vi "SW_Calc_speed_2.vi"(3 "Speed smoothing type":u16(ring)=3 items=["None", "Holoborodko 2/5", "Holoborodko 2/7", "Holoborodko 2/11", "Holoborodko 4/7"], 4 "X coord, mm":dbl, 5 "Y coord, mm":dbl, 6 "Time per frame, s":dbl) -> (2 "Mouse speed, mm/s":dbl)   [LabVIEW 2018]
doc: "This VI calculates speed using smoothing of the input noisy data according to Holoborodko' algorithm: http://www.holoborodko.com/pavel/numerical-methods/numerical-derivative/smooth-low-noise-differentiator"
panel:
  out "Mouse speed for saving, mm/s":string
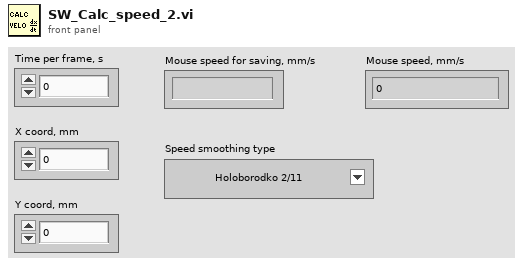
[diagram p1: front panel]
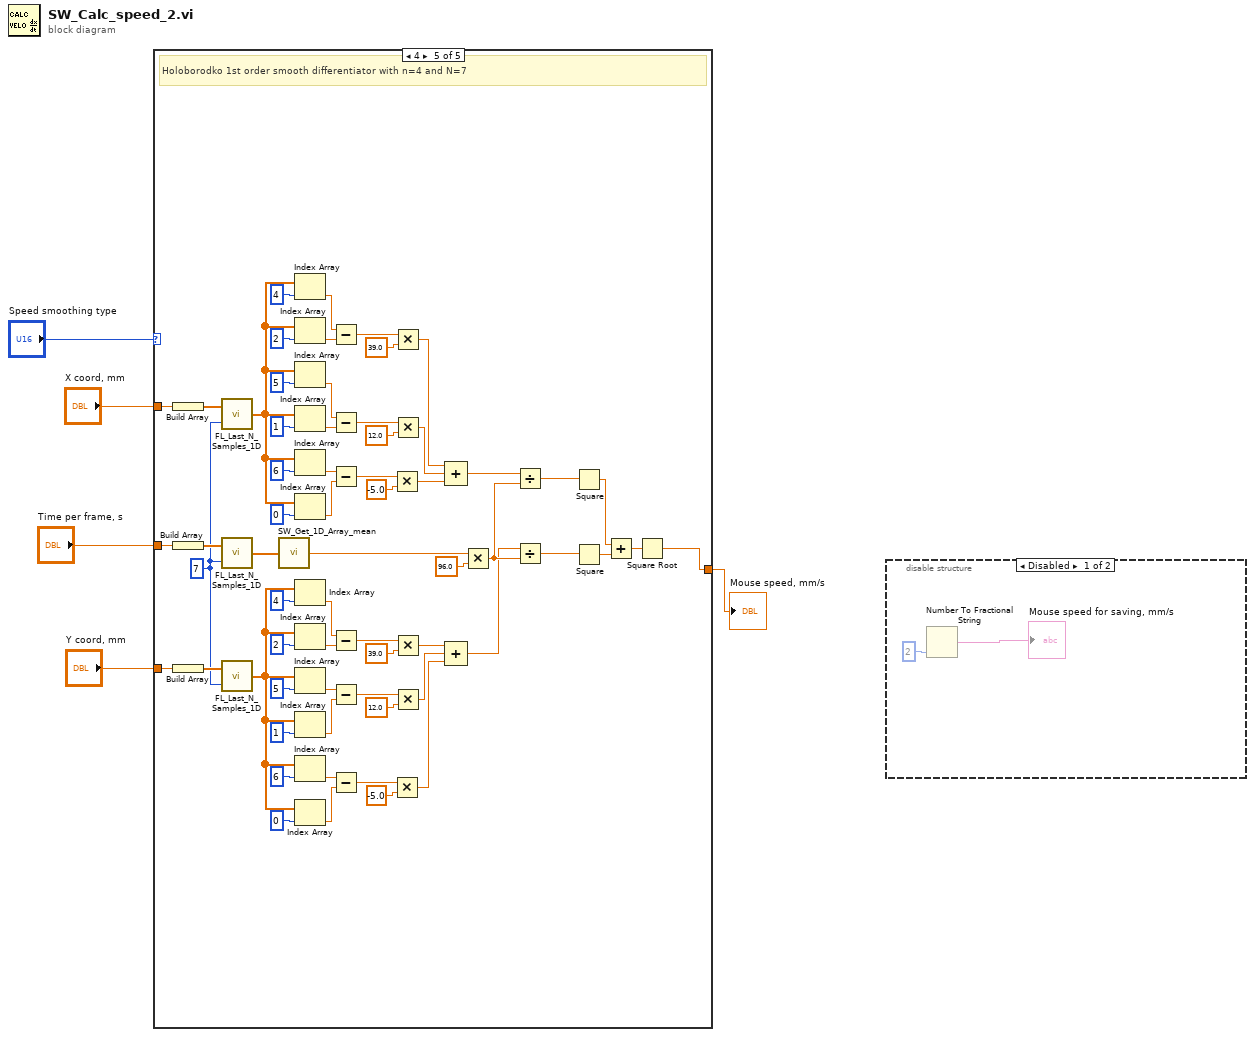
[diagram p0: block diagram]
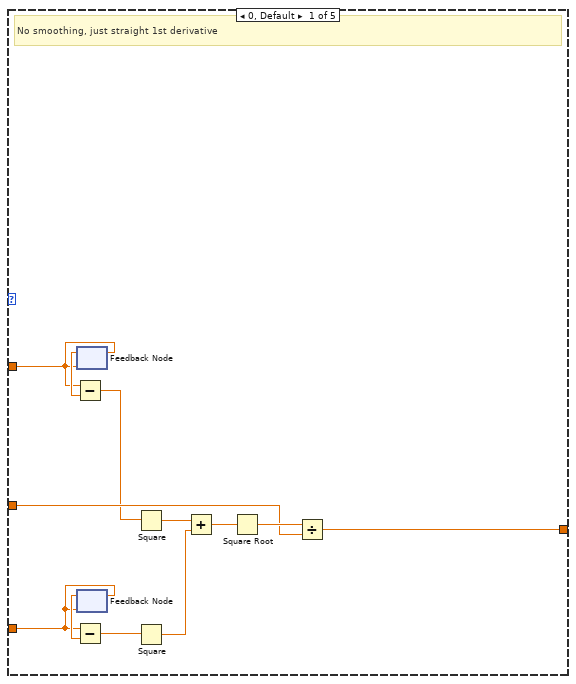
[diagram p3: hidden frame]
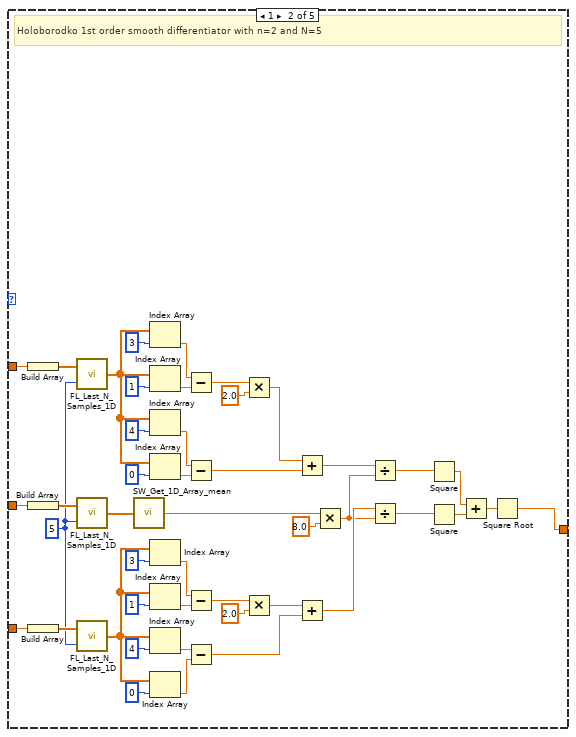
[diagram p4: hidden frame]
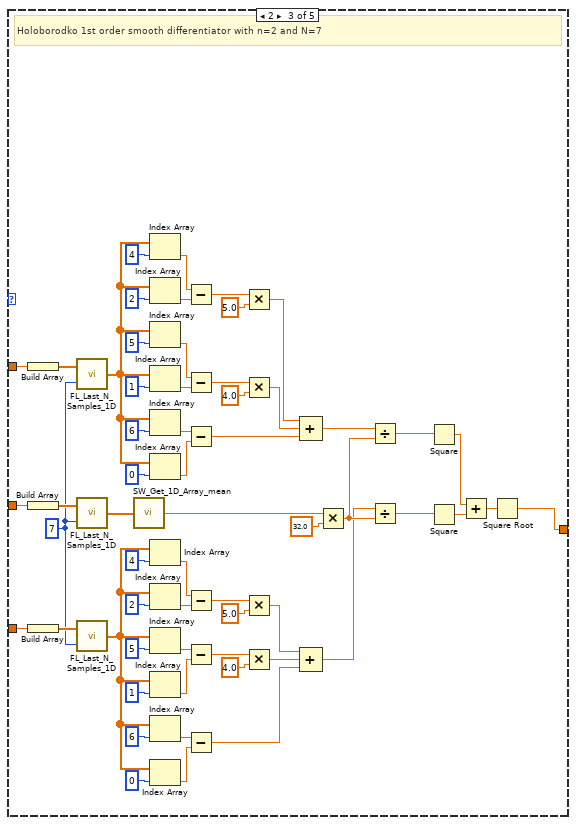
[diagram p5: hidden frame]
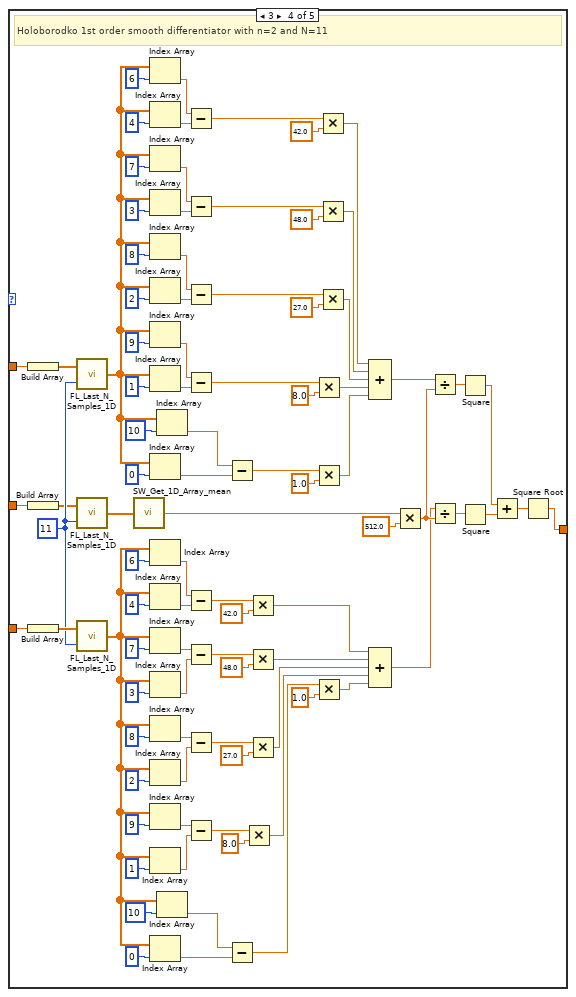
[diagram p6: hidden frame]
diagram:
  n1 = case shown="4" "Speed smoothing type" {
    tunnel: "Time per frame, s" -> [w13 w62 w121 w125 w275]
    tunnel: "Y coord, mm" -> [w7 w58 w117 w210 w271]
    tunnel: "X coord, mm" -> [w9 w57 w116 w209 w270]
    tunnel: [w12 w20 w99 w192 w253] -> w1
    frame 0, Default {
      # "No smoothing, just straight 1st derivative"
      n2 = feedback #1(w9) -> (w10:dbl)
      n3 = Subtract(x=w9, y=w10) -> (x-y=w8:dbl)
      n4 = feedback-in #1(w9) -> ()
      n5 = feedback #2(w7) -> (w11:dbl)
      n6 = Subtract(x=w7, y=w11) -> (x-y=w6:dbl)
      n7 = feedback-in #2(w7) -> ()
      n8 = Square(x=w8) -> (x^2=w16:dbl)
      n9 = Square(x=w6) -> (x^2=w17:dbl)
      n10 = Add(x=w16, y=w17) -> (x+y=w15:dbl)
      n11 = Square Root(x=w15) -> (sqrt(x)=w14:dbl)
      n12 = Divide(x=w14, y=w13) -> (x/y=w12:dbl)
    }
    frame 1 {
      w56 = u32 5 ("BufferLengthSamples")
      # "Holoborodko 1st order smooth differentiator with n=2 and N=5"
      n13 = Build Array(w57) -> (w60:dbl[])
      n14 = Build Array(w62) -> (w61:dbl[])
      n15 = Build Array(w58) -> (w59:dbl[])
      n16 = call "FL_Last_N_Samples_1D.vi"("BufferLengthSamples"=w56, "Input Array"=w60) -> ("Output Array"=w47:dbl[])
      n17 = call "FL_Last_N_Samples_1D.vi"("BufferLengthSamples"=w56, "Input Array"=w61) -> ("Output Array"=w19:dbl[])
      n18 = call "FL_Last_N_Samples_1D.vi"("BufferLengthSamples"=w56, "Input Array"=w59) -> ("Output Array"=w27:dbl[])
      n19 = call "SW_Get_1D_Array_mean.vi"("1D array"=w19) -> ("Mean of 1D Array"=w18:dbl)
      n20 = Index Array(array=w47, index=3) -> (element=w53:dbl)
      n21 = Index Array(array=w47, index=1) -> (element=w52:dbl)
      n22 = Index Array(array=w47, index=4) -> (element=w46:dbl)
      n23 = Index Array(array=w47, index=0) -> (element=w45:dbl)
      n24 = Index Array(array=w27, index=3) -> (element=w30:dbl)
      n25 = Index Array(array=w27, index=1) -> (element=w31:dbl)
      n26 = Index Array(array=w27, index=4) -> (element=w36:dbl)
      n27 = Index Array(array=w27, index=0) -> (element=w37:dbl)
      n28 = Subtract(x=w53, y=w52) -> (x-y=w51:dbl)
      n29 = Subtract(x=w46, y=w45) -> (x-y=w43:dbl)
      n30 = Subtract(x=w30, y=w31) -> (x-y=w32:dbl)
      n31 = Subtract(x=w36, y=w37) -> (x-y=w39:dbl)
      n32 = Multiply(x=w51, y=2.0) -> (x*y=w44:dbl)
      n33 = Multiply(x=w32, y=2.0) -> (x*y=w38:dbl)
      n34 = Add(x=w44, y=w43) -> (x+y=w42:dbl)
      n35 = Add(x=w38, y=w39) -> (x+y=w40:dbl)
      n36 = Multiply(x=w18, y=8.0) -> (x*y=w26:dbl)
      n37 = Divide(x=w42, y=w26) -> (x/y=w23:dbl)
      n38 = Divide(x=w40, y=w26) -> (x/y=w21:dbl)
      n39 = Square(x=w23) -> (x^2=w22:dbl)
      n40 = Square(x=w21) -> (x^2=w24:dbl)
      n41 = Add(x=w22, y=w24) -> (x+y=w25:dbl)
      n42 = Square Root(x=w25) -> (sqrt(x)=w20:dbl)
    }
    frame 2 {
      w115 = u32 7 ("BufferLengthSamples")
      # "Holoborodko 1st order smooth differentiator with n=2 and N=7"
      n43 = Build Array(w116) -> (w119:dbl[])
      n44 = Build Array(w121) -> (w120:dbl[])
      n45 = Build Array(w117) -> (w118:dbl[])
      n46 = call "FL_Last_N_Samples_1D.vi"("BufferLengthSamples"=w115, "Input Array"=w119) -> ("Output Array"=w94:dbl[])
      n47 = call "FL_Last_N_Samples_1D.vi"("BufferLengthSamples"=w115, "Input Array"=w120) -> ("Output Array"=w64:dbl[])
      n48 = call "FL_Last_N_Samples_1D.vi"("BufferLengthSamples"=w115, "Input Array"=w118) -> ("Output Array"=w67:dbl[])
      n49 = call "SW_Get_1D_Array_mean.vi"("1D array"=w64) -> ("Mean of 1D Array"=w63:dbl)
      n50 = Index Array(array=w94, index=4) -> (element=w112:dbl)
      n51 = Index Array(array=w94, index=2) -> (element=w111:dbl)
      n52 = Index Array(array=w94, index=5) -> (element=w108:dbl)
      n53 = Index Array(array=w94, index=1) -> (element=w107:dbl)
      n54 = Index Array(array=w94, index=6) -> (element=w97:dbl)
      n55 = Index Array(array=w94, index=0) -> (element=w98:dbl)
      n56 = Index Array(array=w67, index=4) -> (element=w70:dbl)
      n57 = Index Array(array=w67, index=2) -> (element=w71:dbl)
      n58 = Index Array(array=w67, index=5) -> (element=w74:dbl)
      n59 = Index Array(array=w67, index=1) -> (element=w75:dbl)
      n60 = Index Array(array=w67, index=6) -> (element=w77:dbl)
      n61 = Index Array(array=w67, index=0) -> (element=w76:dbl)
      n62 = Subtract(x=w112, y=w111) -> (x-y=w93:dbl)
      n63 = Subtract(x=w108, y=w107) -> (x-y=w91:dbl)
      n64 = Subtract(x=w97, y=w98) -> (x-y=w89:dbl)
      n65 = Subtract(x=w70, y=w71) -> (x-y=w80:dbl)
      n66 = Subtract(x=w74, y=w75) -> (x-y=w82:dbl)
      n67 = Subtract(x=w77, y=w76) -> (x-y=w84:dbl)
      n68 = Multiply(x=w93, y=5.0) -> (x*y=w87:dbl)
      n69 = Multiply(x=w91, y=4.0) -> (x*y=w88:dbl)
      n70 = Multiply(x=w80, y=5.0) -> (x*y=w86:dbl)
      n71 = Multiply(x=w82, y=4.0) -> (x*y=w85:dbl)
      n72 = Compound Arithmetic op=ADD(w87, w88, w89) -> (w66:dbl)
      n73 = Compound Arithmetic op=ADD(w86, w85, w84) -> (w65:dbl)
      n74 = Multiply(x=w63, y=32.0) -> (x*y=w105:dbl)
      n75 = Divide(x=w66, y=w105) -> (x/y=w102:dbl)
      n76 = Divide(x=w65, y=w105) -> (x/y=w100:dbl)
      n77 = Square(x=w102) -> (x^2=w101:dbl)
      n78 = Square(x=w100) -> (x^2=w103:dbl)
      n79 = Add(x=w101, y=w103) -> (x+y=w104:dbl)
      n80 = Square Root(x=w104) -> (sqrt(x)=w99:dbl)
    }
    frame 3 {
      w208 = u32 11 ("BufferLengthSamples")
      # "Holoborodko 1st order smooth differentiator with n=2 and N=11"
      n81 = Build Array(w209) -> (w212:dbl[])
      n82 = Build Array(w125) -> (w124:dbl[])
      n83 = Build Array(w210) -> (w211:dbl[])
      n84 = call "FL_Last_N_Samples_1D.vi"("BufferLengthSamples"=w208, "Input Array"=w212) -> ("Output Array"=w165:dbl[])
      n85 = call "FL_Last_N_Samples_1D.vi"("BufferLengthSamples"=w208, "Input Array"=w124) -> ("Output Array"=w123:dbl[])
      n86 = call "FL_Last_N_Samples_1D.vi"("BufferLengthSamples"=w208, "Input Array"=w211) -> ("Output Array"=w127:dbl[])
      n87 = call "SW_Get_1D_Array_mean.vi"("1D array"=w123) -> ("Mean of 1D Array"=w122:dbl)
      n88 = Index Array(array=w165, index=6) -> (element=w205:dbl)
      n89 = Index Array(array=w165, index=4) -> (element=w204:dbl)
      n90 = Index Array(array=w165, index=7) -> (element=w201:dbl)
      n91 = Index Array(array=w165, index=3) -> (element=w200:dbl)
      n92 = Index Array(array=w165, index=8) -> (element=w190:dbl)
      n93 = Index Array(array=w165, index=2) -> (element=w191:dbl)
      n94 = Index Array(array=w165, index=9) -> (element=w173:dbl)
      n95 = Index Array(array=w165, index=1) -> (element=w172:dbl)
      n96 = Index Array(array=w165, index=0) -> (element=w171:dbl)
      n97 = Index Array(array=w127, index=6) -> (element=w130:dbl)
      n98 = Index Array(array=w127, index=4) -> (element=w131:dbl)
      n99 = Index Array(array=w127, index=7) -> (element=w134:dbl)
      n100 = Index Array(array=w127, index=3) -> (element=w135:dbl)
      n101 = Index Array(array=w127, index=8) -> (element=w137:dbl)
      n102 = Index Array(array=w127, index=2) -> (element=w136:dbl)
      n103 = Index Array(array=w127, index=9) -> (element=w153:dbl)
      n104 = Index Array(array=w127, index=1) -> (element=w154:dbl)
      n105 = Index Array(array=w127, index=0) -> (element=w155:dbl)
      n106 = Index Array(array=w165, index=10) -> (element=w170:dbl)
      n107 = Index Array(array=w127, index=10) -> (element=w156:dbl)
      n108 = Subtract(x=w205, y=w204) -> (x-y=w187:dbl)
      n109 = Subtract(x=w201, y=w200) -> (x-y=w185:dbl)
      n110 = Subtract(x=w190, y=w191) -> (x-y=w183:dbl)
      n111 = Subtract(x=w173, y=w172) -> (x-y=w176:dbl)
      n112 = Subtract(x=w130, y=w131) -> (x-y=w140:dbl)
      n113 = Subtract(x=w134, y=w135) -> (x-y=w142:dbl)
      n114 = Subtract(x=w137, y=w136) -> (x-y=w144:dbl)
      n115 = Subtract(x=w153, y=w154) -> (x-y=w150:dbl)
      n116 = Subtract(x=w170, y=w171) -> (x-y=w167:dbl)
      n117 = Subtract(x=w156, y=w155) -> (x-y=w159:dbl)
      n118 = Multiply(x=w150, y=8.0) -> (x*y=w161:dbl)
      n119 = Multiply(x=w140, y=42.0) -> (x*y=w146:dbl)
      n120 = Multiply(x=w142, y=48.0) -> (x*y=w145:dbl)
      n121 = Multiply(x=w144, y=27.0) -> (x*y=w147:dbl)
      n122 = Multiply(x=w176, y=8.0) -> (x*y=w164:dbl)
      n123 = Multiply(x=w167, y=1.0) -> (x*y=w163:dbl)
      n124 = Multiply(x=w159, y=1.0) -> (x*y=w162:dbl)
      n125 = Multiply(x=w187, y=42.0) -> (x*y=w181:dbl)
      n126 = Multiply(x=w185, y=48.0) -> (x*y=w182:dbl)
      n127 = Multiply(x=w183, y=27.0) -> (x*y=w179:dbl)
      n128 = Compound Arithmetic op=ADD(w181, w182, w179, w164, w163) -> (w180:dbl)
      n129 = Compound Arithmetic op=ADD(w146, w145, w147, w161, w162) -> (w126:dbl)
      n130 = Multiply(x=w122, y=512.0) -> (x*y=w198:dbl)
      n131 = Divide(x=w180, y=w198) -> (x/y=w195:dbl)
      n132 = Divide(x=w126, y=w198) -> (x/y=w193:dbl)
      n133 = Square(x=w195) -> (x^2=w194:dbl)
      n134 = Square(x=w193) -> (x^2=w196:dbl)
      n135 = Add(x=w194, y=w196) -> (x+y=w197:dbl)
      n136 = Square Root(x=w197) -> (sqrt(x)=w192:dbl)
    }
    frame 4 {
      w269 = u32 7 ("BufferLengthSamples")
      # "Holoborodko 1st order smooth differentiator with n=4 and N=7"
      n137 = Build Array(w270) -> (w273:dbl[])
      n138 = Build Array(w275) -> (w274:dbl[])
      n139 = Build Array(w271) -> (w272:dbl[])
      n140 = call "FL_Last_N_Samples_1D.vi"("BufferLengthSamples"=w269, "Input Array"=w273) -> ("Output Array"=w248:dbl[])
      n141 = call "FL_Last_N_Samples_1D.vi"("BufferLengthSamples"=w269, "Input Array"=w274) -> ("Output Array"=w214:dbl[])
      n142 = call "FL_Last_N_Samples_1D.vi"("BufferLengthSamples"=w269, "Input Array"=w272) -> ("Output Array"=w221:dbl[])
      n143 = call "SW_Get_1D_Array_mean.vi"("1D array"=w214) -> ("Mean of 1D Array"=w213:dbl)
      n144 = Index Array(array=w248, index=4) -> (element=w266:dbl)
      n145 = Index Array(array=w248, index=2) -> (element=w265:dbl)
      n146 = Index Array(array=w248, index=5) -> (element=w262:dbl)
      n147 = Index Array(array=w248, index=1) -> (element=w261:dbl)
      n148 = Index Array(array=w248, index=6) -> (element=w251:dbl)
      n149 = Index Array(array=w248, index=0) -> (element=w252:dbl)
      n150 = Index Array(array=w221, index=4) -> (element=w224:dbl)
      n151 = Index Array(array=w221, index=2) -> (element=w225:dbl)
      n152 = Index Array(array=w221, index=5) -> (element=w228:dbl)
      n153 = Index Array(array=w221, index=1) -> (element=w229:dbl)
      n154 = Index Array(array=w221, index=6) -> (element=w231:dbl)
      n155 = Index Array(array=w221, index=0) -> (element=w230:dbl)
      n156 = Subtract(x=w266, y=w265) -> (x-y=w247:dbl)
      n157 = Subtract(x=w262, y=w261) -> (x-y=w245:dbl)
      n158 = Subtract(x=w251, y=w252) -> (x-y=w243:dbl)
      n159 = Subtract(x=w224, y=w225) -> (x-y=w234:dbl)
      n160 = Subtract(x=w228, y=w229) -> (x-y=w236:dbl)
      n161 = Subtract(x=w231, y=w230) -> (x-y=w238:dbl)
      n162 = Multiply(x=w243, y=-5.0) -> (x*y=w218:dbl)
      n163 = Multiply(x=w238, y=-5.0) -> (x*y=w216:dbl)
      n164 = Multiply(x=w247, y=39.0) -> (x*y=w241:dbl)
      n165 = Multiply(x=w245, y=12.0) -> (x*y=w242:dbl)
      n166 = Multiply(x=w234, y=39.0) -> (x*y=w240:dbl)
      n167 = Multiply(x=w236, y=12.0) -> (x*y=w239:dbl)
      n168 = Compound Arithmetic op=ADD(w241, w242, w218) -> (w220:dbl)
      n169 = Compound Arithmetic op=ADD(w240, w239, w216) -> (w219:dbl)
      n170 = Multiply(x=w213, y=96.0) -> (x*y=w259:dbl)
      n171 = Divide(x=w220, y=w259) -> (x/y=w256:dbl)
      n172 = Divide(x=w219, y=w259) -> (x/y=w254:dbl)
      n173 = Square(x=w256) -> (x^2=w255:dbl)
      n174 = Square(x=w254) -> (x^2=w257:dbl)
      n175 = Add(x=w255, y=w257) -> (x+y=w258:dbl)
      n176 = Square Root(x=w258) -> (sqrt(x)=w253:dbl)
    }
  }
  "Mouse speed, mm/s" <- w1
  n177 = disable-structure shown="Disabled" {
    frame Disabled {
      n178 = Number To Fractional String(precision (6)=i16 2) -> (F-format string=→"Mouse speed for saving, mm/s":string)  [unwired: 3 in]
    }
    frame Enabled {
    }
  }
